vi "initCAN.vi"(4 "error in":errorcluster, 7 "FPGA VI (in)":T1) -> (0 "error out":errorcluster, 1 "CAN":T2, 3 "FPGA VI (out)":T1)   [LabVIEW 2017]
uses:
  <resource>/objmgr/xnet.rc
  <vilib>/xnet/xnet.llb/XNET Create Session (Frame Output Stream).vi
  <vilib>/xnet/xnet.llb/XNET Create Session (Frame Input Stream).vi
  FPGA Bitfiles/FPGA.ctl
panel:
  out "error out 2":errorcluster
  out "iteration":i32
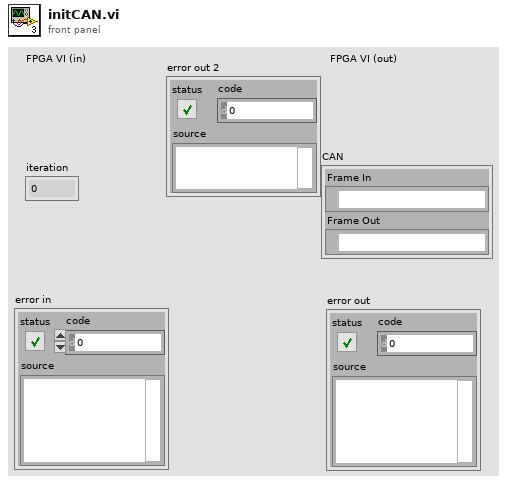
[diagram p1: front panel]
types:
  T1 = typedef "FPGA.ctl" = refnum<k20>
  T2 = cluster{"Frame In":refnum<k21>, "Frame Out":refnum<k21>}
  T3 = cluster{"session out":refnum<k21>, "session out":refnum<k21>}
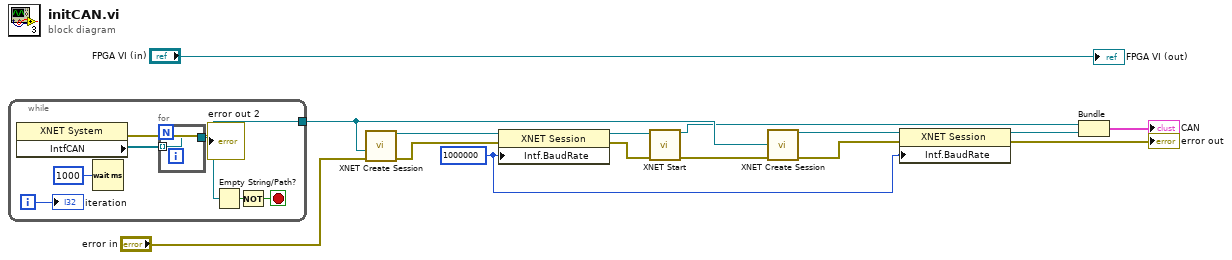
[diagram p0: block diagram]
diagram:
  w8 = u32 1000000 ("y")
  n1 = while {
    tunnel: [w17] -> w7
    i -> [w18]
    stop <- w19 stop-if-true
    n2 = property class="XNET System"() -> (error out=→"error out 2":errorcluster, "IntfCAN"=w22:refnum<k21>[])  [unwired: 2 in, 1 out]
    n3 = Wait (ms)(milliseconds to wait=u32 1000) -> ()  [unwired: 1 out]
    n4 = for {
      tunnel: w22 -> [w23] mode=indexing
      tunnel: [w23] -> w17
    }
    n5 = Empty String/Path?(string/path=w17) -> (empty?=w20:bool)
    n6 = Not(x=w20) -> (.not. x?=w19:bool)
    "iteration" <- w18
  }
  n7 = call-poly <vilib>:"XNET Create Session.vi"("interface"=w7, "error in (no error)"="error in") -> ("session out"=w13:refnum<k21>, "error out"=w14:errorcluster)  [unwired: 1 in, 11 out]
  n8 = property class="XNET Session"(reference=w13, error in=w14, "Intf.BaudRate"=w8) -> (reference out=w12:refnum<k21>, error out=w11:errorcluster)
  n9 = call <vilib>:"XNET Start.vi"("session in"=w12, "error in (no error)"=w11) -> ("session out"=w4:refnum<k21>, "error out"=w10:errorcluster)  [unwired: 12 out]
  n10 = call-poly <vilib>:"XNET Create Session.vi"("interface"=w7, "error in (no error)"=w10) -> ("session out"=w15:refnum<k21>, "error out"=w9:errorcluster)  [unwired: 1 in, 11 out]
  n11 = property class="XNET Session"(reference=w15, error in=w9, "Intf.BaudRate"=w8) -> (reference out=w3:refnum<k21>, error out=→"error out":errorcluster)
  n12 = Bundle("session out"=w4, "session out"=w3) -> (→"CAN":T3)  [unwired: 1 in]
  "FPGA VI (out)" <- "FPGA VI (in)"
